vi "Teleop Winch with Setpoint Control.vi"(3 "error in (no error)":errorcluster, 4 "Joystick Command":dbl, 5 "MotorControlDevRef":T1) -> (0 "error out":errorcluster, 1 "Commanded\nSet Output":dbl, 2 "MotorControlOutput":T1={"DeviceStatus"={"status"=FALSE, "code"=0, "source"=""}, "Type"=enum."PWM", "PWM"={"PWM Channel"=enum."Invalid", "DeadBand"={"Name"="", "maxPositivePwm"=0, "minPositivePwm"=0, "centerPwm"=0, "maxNegativePwm"=0, "minNegativePwm"=0, "angularRange"=0}}, "CAN"={"Device Number"=0, "SetOutput VI Ref"=variant(refnum<vi> refnum), "GetOutput VI Ref"=variant(refnum<vi> refnum), "Enable VI Ref"=variant(refnum<vi> refnum), "Disable VI Ref"=variant(refnum<vi> refnum), "Data"=variant}, "Invert"=FALSE, "DIO PWM"={"PWM \"Enable\" Channel"=enum."Invalid", "DIOChannel"=enum."Invalid", "PWM Rate"=0.0}})   [LabVIEW 2020]
doc: "This takes a value from a joystick, applies a deadband to the value and then multiples the value by 0.2 to get the value to add to the current setpoint."
uses:
  <vilib>/Rock Robotics/WPI/MotorControl/WPI_MotorControlDeviceRef.ctl
  <vilib>/Rock Robotics/WPI/MotorControl/WPI_MotorControlType.ctl
  <vilib>/Rock Robotics/SystemInterfaces/DIO/FPGA_DIOPWMChannel.ctl
  <vilib>/Rock Robotics/WPI/PWM/WPI_PWMDeadband.ctl
  <vilib>/Rock Robotics/SystemInterfaces/DIO/FPGA_DIOChannel.ctl
  <vilib>/Rock Robotics/WPI/ThirdParty/REV Robotics/REVLib/Typedef/Spark MAX Control Type.ctl
  2022 Robot Global Data.vi
panel:
  out "Error\n(armSetpoint -\n armPosition)":dbl
  out "Premove\nSensor Position":dbl
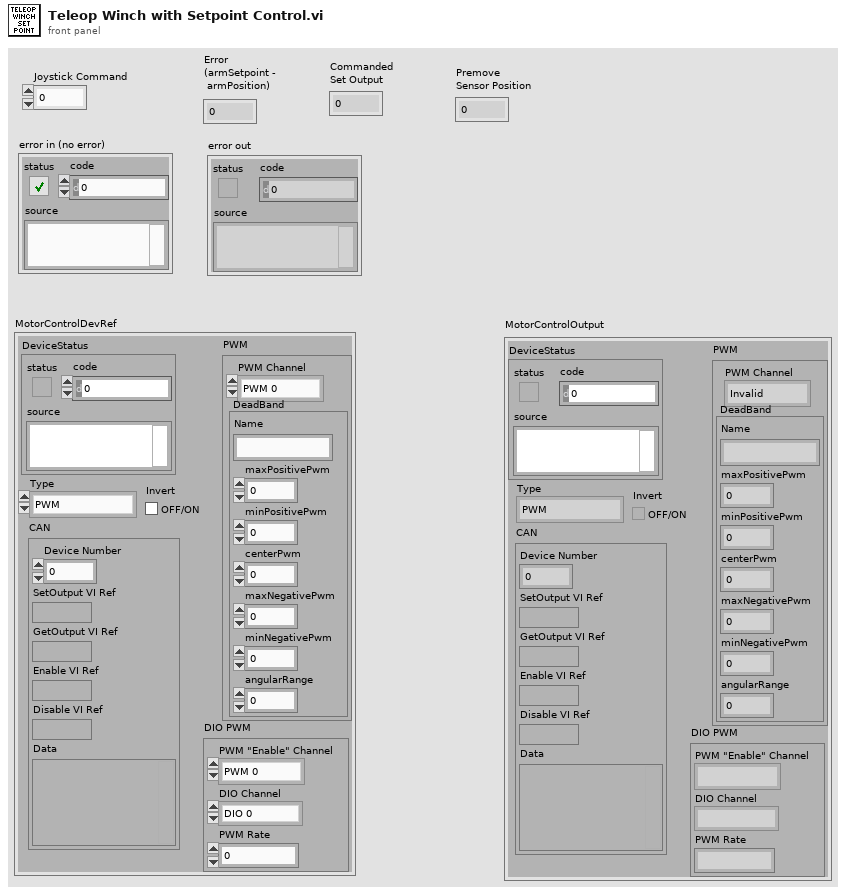
[diagram p1: front panel]
types:
  T1 = typedef "WPI_MotorControlDeviceRef.ctl" = cluster{"DeviceStatus":errorcluster, "Type":T2, "PWM":cluster{"PWM Channel":T3, "DeadBand":T4}, "CAN":cluster{"Device Number":u8, "SetOutput VI Ref":variant, "GetOutput VI Ref":variant, "Enable VI Ref":variant, "Disable VI Ref":variant, "Data":variant}, "Invert":bool, "DIO PWM":cluster{"PWM \"Enable\" Channel":T3, "DIOChannel":T5, "PWM Rate":dbl}}
  T2 = typedef "WPI_MotorControlType.ctl" = enum16{"PWM", "CAN", "DIO PWM"}
  T3 = typedef "FPGA_DIOPWMChannel.ctl" = enum8{"PWM 0", "PWM 1", "PWM 2", "PWM 3", "PWM 4", "PWM 5", "PWM 6", "PWM 7", "PWM 8", "PWM 9", "PWM MXP 0", "PWM MXP 1", "PWM MXP 2", "PWM MXP 3", "PWM MXP 4", "PWM MXP 5", "PWM MXP 6", "PWM MXP 7", "PWM MXP 8", "PWM MXP 9", "Invalid"}
  T4 = typedef "WPI_PWMDeadband.ctl" = cluster{"Name":string, "maxPositivePwm":i32, "minPositivePwm":i32, "centerPwm":i32, "maxNegativePwm":i32, "minNegativePwm":i32, "angularRange":u16}
  T5 = typedef "FPGA_DIOChannel.ctl" = enum8{"DIO 0", "DIO 1", "DIO 2", "DIO 3", "DIO 4", "DIO 5", "DIO 6", "DIO 7", "DIO 8", "DIO 9", "DIO MXP 0", "DIO MXP 1", "DIO MXP 2", "DIO MXP 3", "DIO MXP 4", "DIO MXP 5", "DIO MXP 6", "DIO MXP 7", "DIO MXP 8", "DIO MXP 9", "DIO MXP 10", "DIO MXP 11", "DIO MXP 12", "DIO MXP 13", "DIO MXP 14", "DIO MXP 15", "SPI Port CS1", "SPI Port CS2", "SPI Port CS3", "SPI Port MISO", "SPI Port MOSI", "Invalid"}
  T6 = typedef "Spark MAX Control Type.ctl" = enum16{"Percent VBus", "Voltage", "Velocity", "Position", "Smart Motion", "Current", "Smart Velocity"}
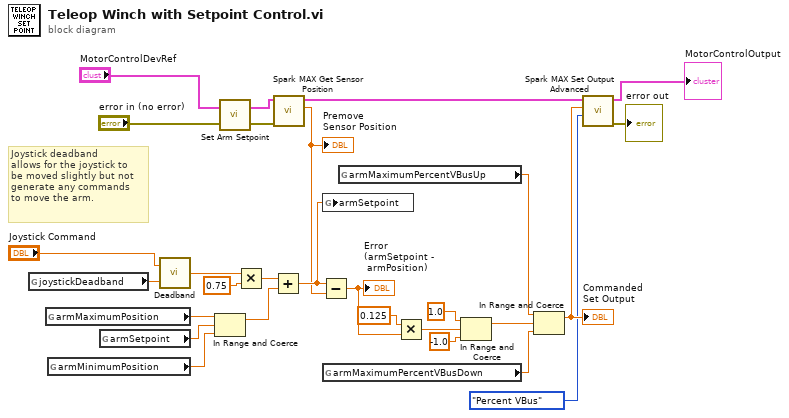
[diagram p0: block diagram]
diagram:
  # "Joystick deadband\nallows for the joystick to\nbe moved slightly but not\ngenerate any commands\nto move the arm."
  n1 = global read "2022 Robot Global Data.vi" "joystickDeadband"() -> (w1:dbl)
  n2 = global read "2022 Robot Global Data.vi" "armMaximumPosition"() -> (w8:dbl)
  n3 = global read "2022 Robot Global Data.vi" "armMinimumPosition"() -> (w7:dbl)
  n4 = global read "2022 Robot Global Data.vi" "armSetpoint"() -> (w9:dbl)
  n5 = call "Deadband.vi"("Limit"=w1, "Input"="Joystick Command") -> ("Output"=w6:dbl)
  n6 = In Range and Coerce(upper limit=w8, x=w9, lower limit=w7) -> (coerced(x)=w11:dbl)  [unwired: 1 out]
  n7 = call "Set Arm Setpoint.vi"("error in (no error)"="error in (no error)", "MotorControlDevRef in"="MotorControlDevRef") -> ("error out"=w27:errorcluster, "MotorControlDevRef out"=w24:T1)
  n8 = Multiply(x=w6, y=0.75) -> (x*y=w10:dbl)
  n9 = Add(x=w10, y=w11) -> (x+y=w18:dbl)
  n10 = call <vilib>:"Spark MAX Get Sensor Position.vi"("error in (no error)"=w27, "MotorControlDevRef in"=w24) -> ("Sensor Position"=w17:dbl, "MotorControlDevRef out"=w19:T1)  [unwired: 6 in, 2 out]
  "Premove\nSensor Position" <- w17
  n11 = Subtract(x=w18, y=w17) -> (x-y=w12:dbl)
  "Error\n(armSetpoint -\n armPosition)" <- w12
  n12 = global write "2022 Robot Global Data.vi" "armSetpoint"(w18) -> ()
  n13 = global read "2022 Robot Global Data.vi" "armMaximumPercentVBusDown"() -> (w2:dbl)
  n14 = global read "2022 Robot Global Data.vi" "armMaximumPercentVBusUp"() -> (w22:dbl)
  n15 = Multiply(x=0.125, y=w12) -> (x*y=w15:dbl)
  n16 = In Range and Coerce(upper limit=1.0, x=w15, lower limit=-1.0) -> (coerced(x)=w20:dbl)  [unwired: 1 out]
  n17 = In Range and Coerce(upper limit=w22, x=w20, lower limit=w2) -> (coerced(x)=w28:dbl)  [unwired: 1 out]
  "Commanded\nSet Output" <- w28
  n18 = call <vilib>:"Spark MAX Set Output Advanced.vi"("Control Mode"=Spark_MAX_Control_Type."Percent VBus", "Setpoint"=w28, "MotorControlDevRef"=w19) -> ("error out"=→"error out":errorcluster, "MotorControlDevRef"=→"MotorControlOutput":T1)  [unwired: 7 in]
